vi "Load SS Safety.vi"(8 "Ball Gatherer State":T1=enum."Positional", 10 "Load Actuator Values In":T2) -> (2 "Load Actuator Values Out":T2)   [LabVIEW 2015]
uses:
  Load Actuator Values.ctl
  Ball Gatherer State.ctl
  Global Variables/Sensor Data.vi
  Global Variables/Settings.vi
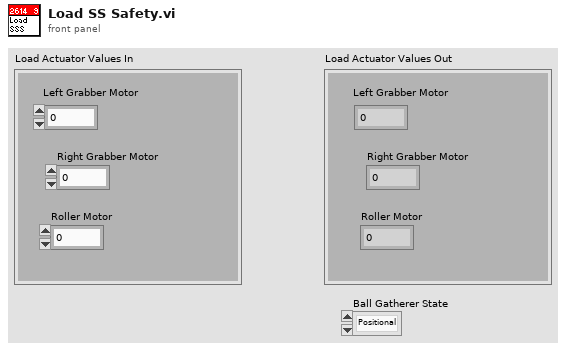
[diagram p1: front panel]
types:
  T1 = typedef "Ball Gatherer State.ctl" = enum16{"Manual", "Positional"}
  T2 = typedef "Load Actuator Values.ctl" = cluster{"Left Grabber Motor":dbl, "Right Grabber Motor":dbl, "Roller Motor":dbl}
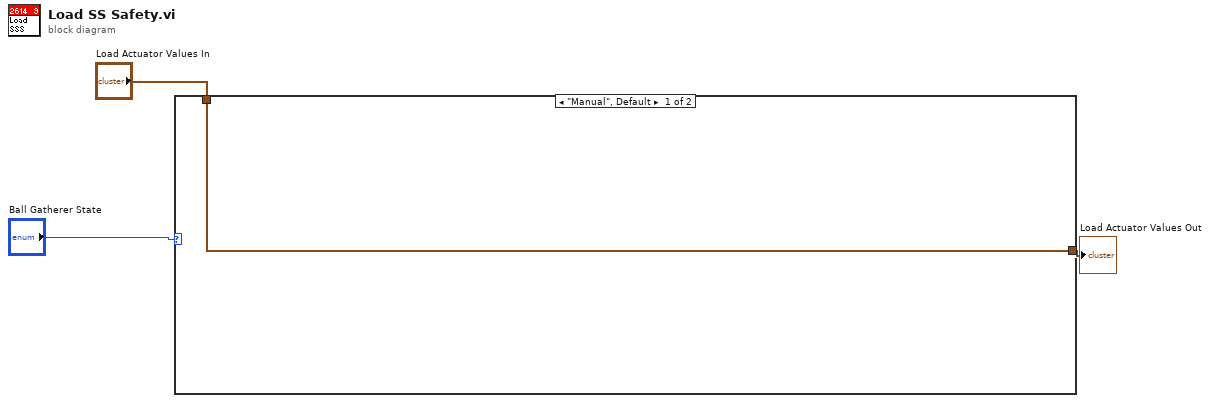
[diagram p0: block diagram]
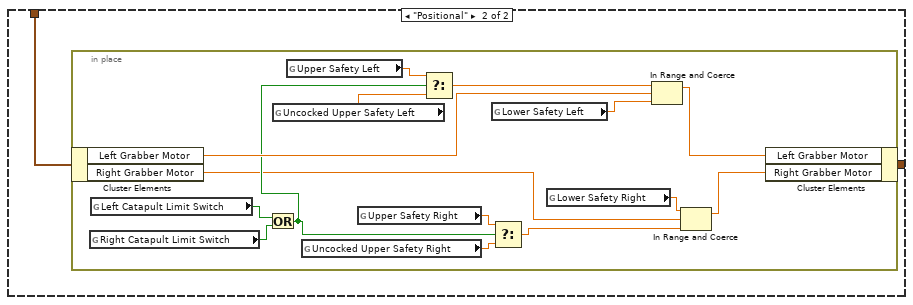
[diagram p2: hidden frame]
diagram:
  n1 = case shown="\"Manual\", Default" "Ball Gatherer State" {
    tunnel: [w4 w6] -> w3
    tunnel: "Load Actuator Values In" -> [w4 w5]
    frame "Manual", Default {
    }
    frame "Positional" {
      n2 = in-place {
        n3 = in-place-cluster #1(w5) -> ("Left Grabber Motor"=w20:dbl, "Right Grabber Motor"=w10:dbl)
        n4 = global read "Sensor Data.vi" "Right Catapult Limit Switch"() -> (w16:bool)
        n5 = global read "Sensor Data.vi" "Left Catapult Limit Switch"() -> (w15:bool)
        n6 = Or(x=w15, y=w16) -> (x .or. y?=w14:bool)
        n7 = global read "Settings.vi" "Uncocked Upper Safety Left"() -> (w13:dbl)
        n8 = global read "Settings.vi" "Upper Safety Left"() -> (w12:dbl)
        n9 = global read "Settings.vi" "Uncocked Upper Safety Right"() -> (w7:dbl)
        n10 = global read "Settings.vi" "Upper Safety Right"() -> (w8:dbl)
        n11 = Select(t=w12, s=w14, f=w13) -> (s? t:f=w21:dbl)
        n12 = global read "Settings.vi" "Lower Safety Left"() -> (w11:dbl)
        n13 = Select(t=w8, s=w14, f=w7) -> (s? t:f=w18:dbl)
        n14 = global read "Settings.vi" "Lower Safety Right"() -> (w9:dbl)
        n15 = In Range and Coerce(upper limit=w21, x=w20, lower limit=w11) -> (coerced(x)=w19:dbl)  [unwired: 1 out]
        n16 = In Range and Coerce(upper limit=w9, x=w10, lower limit=w18) -> (coerced(x)=w17:dbl)  [unwired: 1 out]
        n17 = in-place-cluster #1("Left Grabber Motor"=w19, "Right Grabber Motor"=w17) -> (w6:T2)
      }
    }
  }
  "Load Actuator Values Out" <- w3
